vi "Write to Log File camera.vi"(8 "error in (no error)":errorcluster, 10 "AVI Refnum in":T2, 11 "Array":T1[](array[typedef])) -> (0 "error out":errorcluster, 3 "AVI Refnum output":T2)   [LabVIEW 2017]
uses:
  <vilib>/vision/Avi.llb/IMAQ AVI2 Refnum.ctl
  <vilib>/vision/Image Controls.llb/IMAQ Image.ctl
  <vilib>/vision/Avi.llb/IMAQ AVI2 Codec Path.ctl
panel:
  out "Array 2":T1[](array[typedef])
  out "Webcam":T1(plugin-control)
  out "Codec Names":string[](array[string])
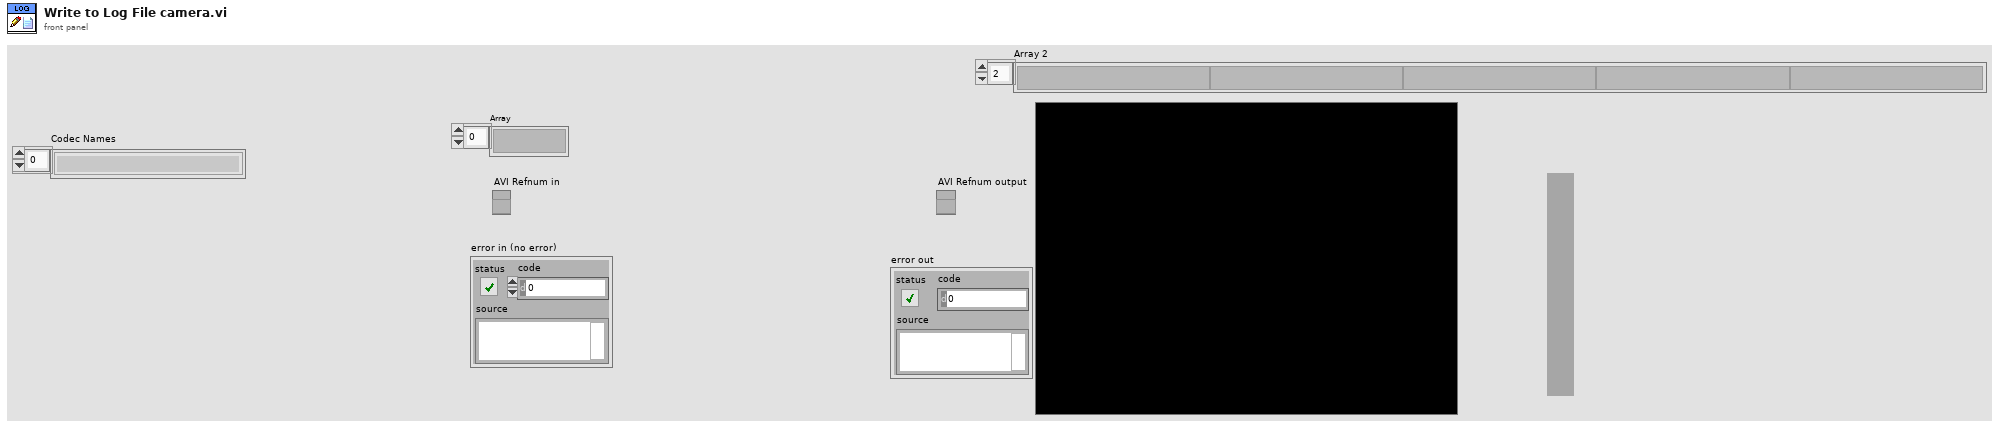
[diagram p1: front panel]
types:
  T1 = typedef "IMAQ Image.ctl" = refnum<image>
  T2 = typedef "IMAQ AVI2 Refnum.ctl" = refnum<k20>
  T3 = typedef "IMAQ AVI2 Codec Path.ctl" = u32
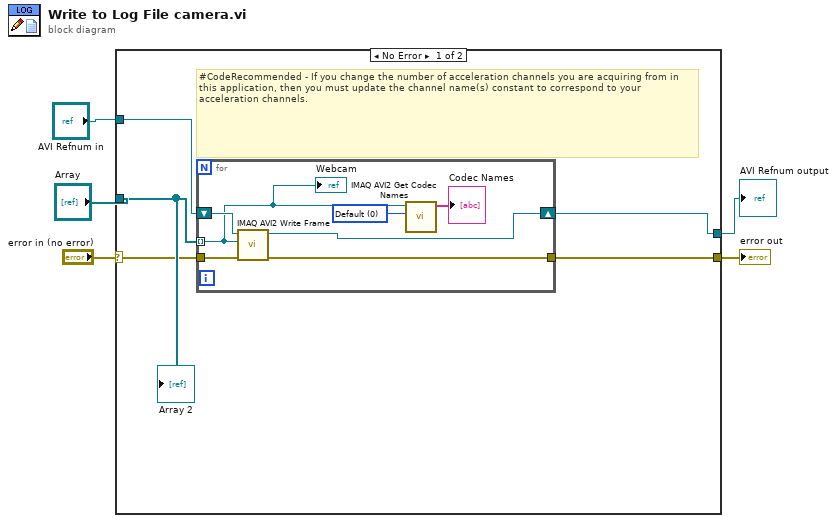
[diagram p0: block diagram]
diagram:
  n1 = case shown="No Error" "error in (no error)" {
    selector: "error in (no error)" -> [w7 w19]
    tunnel: [w6 w19] -> w1
    tunnel: [w8 w18] -> w4
    tunnel: "Array" -> [w10 _]
    tunnel: "AVI Refnum in" -> [w9 w18]
    frame No Error {
      # "#CodeRecommended - If you change the number of acceleration channels you are acquiring from in this application, then you must update the channel name(s) constant to correspond to your acceleration channels."
      n2 = for {
        tunnel: w10 -> [w11] mode=indexing
        tunnel: w7 -> [w15]
        tunnel: [w14] -> w6
        shift-right: [w16] -> w8
        shift-left: w9 -> [w17]
        w13 = T3 0 items=["Default", "System", "Built in Vision"] ("Codec Source")
        n3 = call "IMAQ AVI2 Write Frame"("error in (no error)"=w15, "Image"=w11, "AVI Refnum"=w17) -> ("error out"=w14:errorcluster, "AVI Refnum (duplicate)"=w16:T2)  [unwired: 6 in, 1 out]
        n4 = call "IMAQ AVI2 Get Codec Names"("Codec Source"=w13, "Image"=w11) -> ("Codec Names"=→"Codec Names":string[])  [unwired: 8 in, 1 out]
        "Webcam" <- w11
      }
      "Array 2" <- w10
    }
    frame Error {
    }
  }
  "error out" <- w1
  "AVI Refnum output" <- w4
